vi "DraggingDresser.vi"() -> ()   [LabVIEW 2015]
panel:
  out "Force":dbl[](array[numeric])
  out "Angle for Minimum Force":i32 format="%.1f"
  in  "Coefficient of Kinetic Friction":dbl format="%.1f"
  out "Waveform Graph":dbl[](graph)
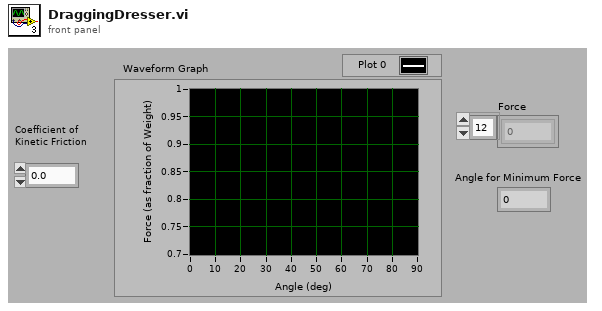
[diagram p1: front panel]
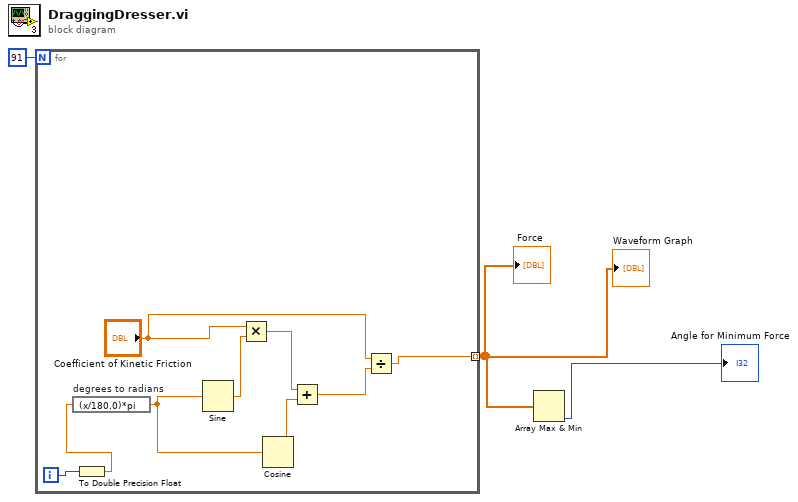
[diagram p0: block diagram]
diagram:
  n1 = for {
    N: 91 -> [_]
    tunnel: [w4] -> w1 mode=indexing
    i -> [w7]
    n2 = To Double Precision Float(number=w7) -> (double precision float=w6:dbl)
    n3 = expression code="(x/180.0)*pi" "degrees to radians"(w6) -> (w5:dbl)
    n4 = Sine(x=w5) -> (sin(x)=w12:dbl)
    n5 = Multiply(x="Coefficient of Kinetic Friction", y=w12) -> (x*y=w11:dbl)
    n6 = Cosine(x=w5) -> (cos(x)=w10:dbl)
    n7 = Add(x=w11, y=w10) -> (x+y=w8:dbl)
    n8 = Divide(x="Coefficient of Kinetic Friction", y=w8) -> (x/y=w4:dbl)
  }
  "Waveform Graph" <- w1
  "Force" <- w1
  n9 = Array Max & Min(array=w1) -> (min index (indices)=→"Angle for Minimum Force":i32)  [unwired: 3 out]
